vi "Read AutoSizeRowsMode.vi"(8 "error in (no error)":errorcluster, 11 "DataGridView in":refnum<class "DataGridView.lvclass">) -> (0 "error out":errorcluster, 2 "AutoSizeRowsMode":i32(ring)=11 items=["None"=0, "AllHeaders"=5, "AllCellsExceptHeaders"=6, "AllCells"=7, "DisplayedHeaders"=9, "DisplayedCellsExceptHeaders"=10, "DisplayedCells"=11], 3 "DataGridView out":refnum<class "DataGridView.lvclass">)   [LabVIEW 2014, in "DataGridView.lvclass"]
uses:
  DataGridView.lvclass
  DataGridView.lvclass/DataGridView.ctl
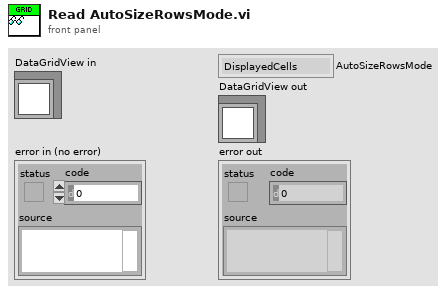
[diagram p1: front panel]
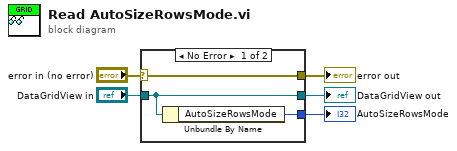
[diagram p0: block diagram]
diagram:
  n1 = case shown="No Error" "error in (no error)" {
    selector: "error in (no error)" -> [w8 w9]
    tunnel: [w8 w9] -> w4
    tunnel: [w7 w10] -> w2
    tunnel: "DataGridView in" -> [w7 w10]
    tunnel: [w6 _] -> w1
    frame No Error {
      n2 = Unbundle By Name(w7) -> ("AutoSizeRowsMode"=w6:i32)
    }
    frame Error {
    }
  }
  "error out" <- w4
  "DataGridView out" <- w2
  "AutoSizeRowsMode" <- w1
